vi "Stiffness and Mass.vi"(4 "k":dbl, 7 "Triangulation In":i32[][](array[numeric]), 10 "Y":dbl[](array[numeric]), 11 "X":dbl[](array[numeric])) -> (2 "Mass Out":T1, 3 "Stiffness Out":T1, 5 "Triangulation Out":i32[][](array[numeric]))   [LabVIEW 2020, in "Heat Equation Solver.lvlib"]
uses:
  Heat Equation Solver.lvlib
  <vilib>/Analysis/Matrix/Datatypes/RealMatrix.ctl
  <vilib>/gmath/NI_PDE.lvlib
  <vilib>/Analysis/Matrix/NI_Matrix.lvlib
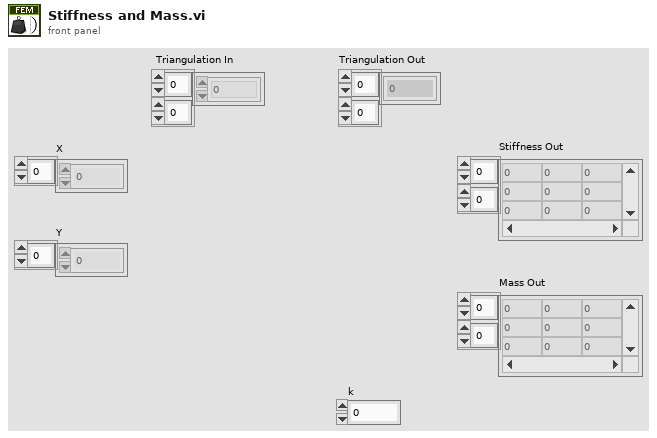
[diagram p1: front panel]
types:
  T1 = typedef "NI_Matrix.lvlib/RealMatrix.ctl" = dbl[][]
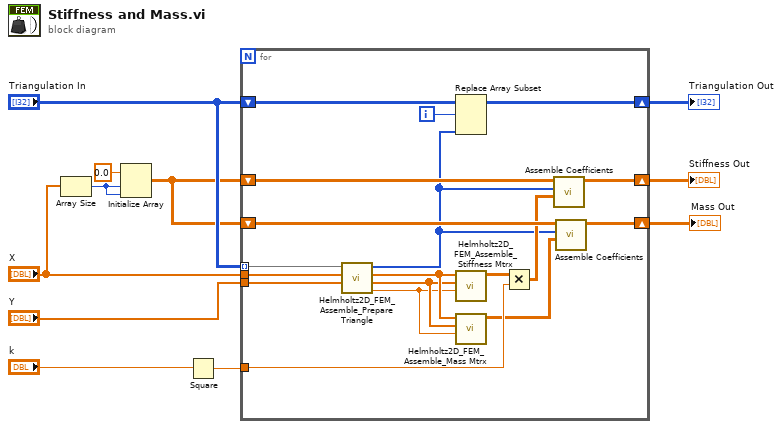
[diagram p0: block diagram]
diagram:
  n1 = Array Size(array="X") -> (size(s)=w2:i32)
  n2 = Initialize Array(0.0 ("element"), w2, w2) -> (w3:dbl[][])
  n3 = Square(x="k") -> (x^2=w11:dbl)
  n4 = for {
    tunnel: "Triangulation In" -> [w21] mode=indexing
    tunnel: "X" -> [w29]
    shift-right: [w26] -> w10
    shift-left: "Triangulation In" -> [w27]
    tunnel: "Y" -> [w28]
    shift-right: [w24] -> w9
    shift-left: w3 -> [w22]
    tunnel: w11 -> [w23]
    shift-right: [w19] -> w5
    shift-left: w3 -> [w20]
    i -> [w25]
    n5 = call <vilib>:"Helmholtz2D_FEM_Assemble_Prepare Triangle.vi"("Y"=w28, "X"=w29, "Triangle In"=w21) -> ("area"=w16:dbl, "Tri Y"=w17:dbl[], "Tri X"=w18:dbl[], "Triangle Out"=w13:i32[])  [unwired: 5 out]
    n6 = Replace Array Subset(array=w27, new element=w13, index (row)=w25) -> (w26:i32[][])  [unwired: 1 in]
    n7 = call <vilib>:"Helmholtz2D_FEM_Assemble_Stiffness Mtrx.vi"("area"=w16, "Tri Y"=w17, "Tri X"=w18) -> ("Stiffness Mtrx"=w15:dbl[][])  [unwired: 8 out]
    n8 = call <vilib>:"Helmholtz2D_FEM_Assemble_Mass Mtrx.vi"("area"=w16, "Tri Y"=w17, "Tri X"=w18) -> ("Mass Mtrx"=w12:dbl[][])  [unwired: 8 out]
    n9 = Multiply(x=w15, y=w23) -> (x*y=w14:dbl[][])
    n10 = call "Assemble Coefficients.vi"("Mtrx"=w14, "Triangle"=w13, "Sparse Matrix In"=w22) -> ("Sparse Matrix Out"=w24:T1)  [unwired: 8 in]
    n11 = call "Assemble Coefficients.vi"("Mtrx"=w12, "Triangle"=w13, "Sparse Matrix In"=w20) -> ("Sparse Matrix Out"=w19:T1)  [unwired: 8 in]
  }
  "Stiffness Out" <- w9
  "Triangulation Out" <- w10
  "Mass Out" <- w5
